vi "Start Stop Temperature Cycle.vi"(8 "error in (no error)":errorcluster, 10 "Start/Stop Cycle":bool, 11 "Temperature Control in":refnum<class "Temperature Control.lvclass">) -> (0 "error out":errorcluster, 2 "Set Point":T1, 3 "Temperature Control out":refnum<class "Temperature Control.lvclass">)   [LabVIEW 2020, in "Temperature Control.lvclass"]
doc: "Start or stop temprature cycle"
uses:
  Temperature Control.lvclass
  Controls/Set point.ctl
  Temperature Control.lvclass/Temperature Control.ctl
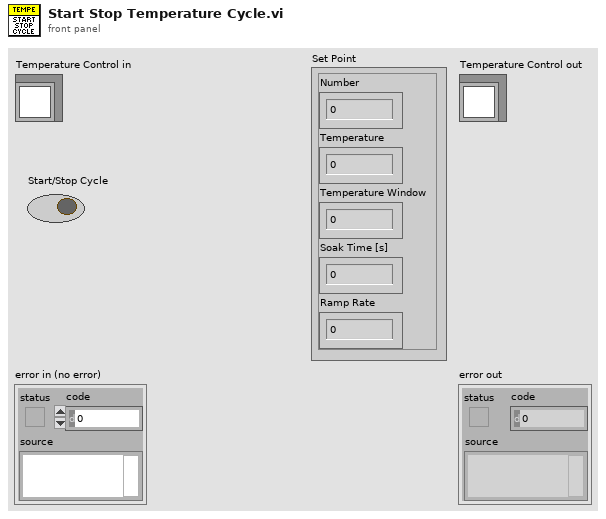
[diagram p1: front panel]
types:
  T1 = typedef "Temperature Control.lvclass/Set point.ctl" = cluster{"Number":u32, "Temperature":dbl, "Temperature Window":dbl, "Soak Time [s]":u32, "Ramp Rate":dbl}
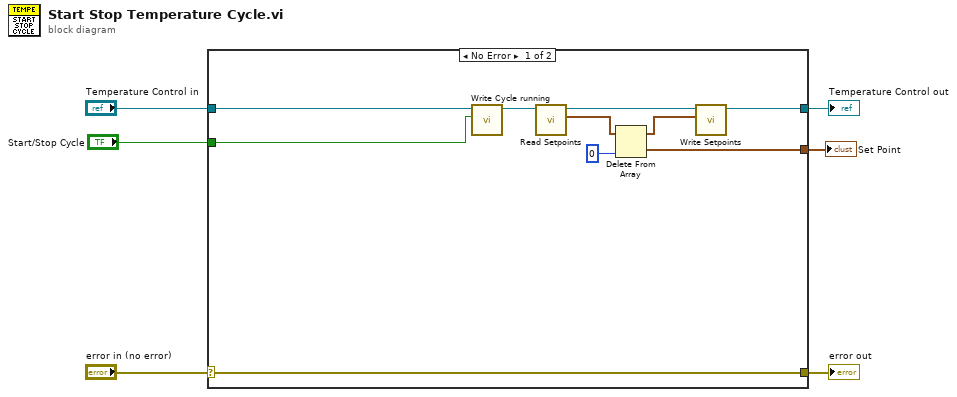
[diagram p0: block diagram]
diagram:
  n1 = case shown="No Error" "error in (no error)" {
    selector: "error in (no error)" -> [w16 w18]
    tunnel: [w16 w18] -> w5
    tunnel: [w11 w17] -> w3
    tunnel: "Temperature Control in" -> [w15 w17]
    tunnel: "Start/Stop Cycle" -> [w14 _]
    tunnel: [w7 _] -> w1
    frame No Error {
      n2 = call "Write Cycle running.vi"("Cycle running"=w14, "Temperature Control in"=w15) -> ("Temperature Control out"=w13:refnum<class "Temperature Control.lvclass">)  [unwired: 9 in]
      n3 = call "Read Setpoints.vi"("Temperature Control in"=w13) -> ("Setpoints"=w10:T1[], "Temperature Control out"=w12:refnum<class "Temperature Control.lvclass">)  [unwired: 9 in]
      n4 = Delete From Array(array=w10, index=0) -> (deleted portion=w7:T1, array with subset deleted=w8:T1[])  [unwired: 1 in]
      n5 = call "Write Setpoints.vi"("Setpoints"=w8, "Temperature Control in"=w12) -> ("Temperature Control out"=w11:refnum<class "Temperature Control.lvclass">)  [unwired: 9 in]
    }
    frame Error {
    }
  }
  "error out" <- w5
  "Temperature Control out" <- w3
  "Set Point" <- w1
